vi "Initialization_channels.vi"(8 "error in (no error)":errorcluster, 9 "productNum":u32, 10 "vendorNum":u32, 11 "Device Item Ref in":T3 format="%.0x") -> (0 "error out":errorcluster, 2 "PAR":T1={"Loop time"={"Loop Rate"=5, "Processor"=-2}, "COM"={"COM IP"="192.168.8.70", "COM port"=30005, "Local port"=5556, "Next_IP 1"=0, "Next_IP 2"=0, "Next_IP 3"=0, "Next_IP 4"=0}, "O2Sensor1"={"Lambda"={"LSU4.2 Lambda"=[], "LSU4.2 Ip"=[], "LSU4.9 Lambda"=[], "LSU4.9 Ip"=[], "LZA03 Lambda"=[], "LZA03 Ip"=[], "LZA08 Lambda"=[], "LZA08 Ip"=[], "Custom Lambda"=[], "Custom Ip"=[]}, "Temp"={"LSU4.2 Temp"=[], "LSU4.2 Ohm"=[], "LSU4.9 Temp"=[], "LSU4.9 Ohm"=[], "LZA03 Temp"=[], "LZA03 Ohm"=[], "LZA08 Temp"=[], "LZA08 Ohm"=[], "Custom Temp"=[], "Custom Ohm"=[]}, "Lambda Type"=0, "PID"={"Ki"=0.0, "Kp"=0.0, "Kd"=0.0, "FeedFW"=0.0}}, "O2Sensor2"={"Lambda"={"LSU4.2 Lambda"=[], "LSU4.2 Ip"=[], "LSU4.9 Lambda"=[], "LSU4.9 Ip"=[], "LZA03 Lambda"=[], "LZA03 Ip"=[], "LZA08 Lambda"=[], "LZA08 Ip"=[], "Custom Lambda"=[], "Custom Ip"=[]}, "Temp"={"LSU4.2 Temp"=[], "LSU4.2 Ohm"=[], "LSU4.9 Temp"=[], "LSU4.9 Ohm"=[], "LZA03 Temp"=[], "LZA03 Ohm"=[], "LZA08 Temp"=[], "LZA08 Ohm"=[], "Custom Temp"=[], "Custom Ohm"=[]}, "Lambda Type"=0, "PID"={"Ki"=0.0, "Kp"=0.0, "Kd"=0.0, "FeedFW"=0.0}}, "O2Sensor3"={"Lambda"={"LSU4.2 Lambda"=[], "LSU4.2 Ip"=[], "LSU4.9 Lambda"=[], "LSU4.9 Ip"=[], "LZA03 Lambda"=[], "LZA03 Ip"=[], "LZA08 Lambda"=[], "LZA08 Ip"=[], "Custom Lambda"=[], "Custom Ip"=[]}, "Temp"={"LSU4.2 Temp"=[], "LSU4.2 Ohm"=[], "LSU4.9 Temp"=[], "LSU4.9 Ohm"=[], "LZA03 Temp"=[], "LZA03 Ohm"=[], "LZA08 Temp"=[], "LZA08 Ohm"=[], "Custom Temp"=[], "Custom Ohm"=[]}, "Lambda Type"=0, "PID"={"Ki"=0.0, "Kp"=0.0, "Kd"=0.0, "FeedFW"=0.0}}, "O2Sensor4"={"Lambda"={"LSU4.2 Lambda"=[], "LSU4.2 Ip"=[], "LSU4.9 Lambda"=[], "LSU4.9 Ip"=[], "LZA03 Lambda"=[], "LZA03 Ip"=[], "LZA08 Lambda"=[], "LZA08 Ip"=[], "Custom Lambda"=[], "Custom Ip"=[]}, "Temp"={"LSU4.2 Temp"=[], "LSU4.2 Ohm"=[], "LSU4.9 Temp"=[], "LSU4.9 Ohm"=[], "LZA03 Temp"=[], "LZA03 Ohm"=[], "LZA08 Temp"=[], "LZA08 Ohm"=[], "Custom Temp"=[], "Custom Ohm"=[]}, "Lambda Type"=0, "PID"={"Ki"=0.0, "Kp"=0.0, "Kd"=0.0, "FeedFW"=0.0}}, "Board"=1, "Mode"=enum."SLSC Mode", "vendor.Num"=4141, "product.Num"=0} {"Board" items=["ALMA-10201", "ALMA-10401"]; "O2Sensor4"."Lambda Type" items=["LSU4.2", "LSU4.9", "LZA03", "LZA08", "Custom", "[mA]"]; "O2Sensor3"."Lambda Type" items=["LSU4.2", "LSU4.9", "LZA03", "LZA08", "Custom", "[mA]"]; "O2Sensor2"."Lambda Type" items=["LSU4.2", "LSU4.9", "LZA03", "LZA08", "Custom", "[mA]"]; "O2Sensor1"."Lambda Type" items=["LSU4.2", "LSU4.9", "LZA03", "LZA08", "Custom", "[mA]"]}, 3 "Device Item Ref out":T3 format="%.0x")   [LabVIEW 2017, in "ALMA_10201-10401_O2SensorSim System Explorer.lvlib"]
uses:
  ALMA_10201-10401_O2SensorSim System Explorer.lvlib
  <vilib>/NI Veristand/Custom Device API/Custom Device Item Ref.ctl
  Engine/Par.ctl
  Engine/LambdaType.ctl
  <vilib>/NI Veristand/Custom Device API/Custom Device Channel.ctl
  <vilib>/NI Veristand/Custom Device API/Custom Device Channel Type.ctl
  <vilib>/NI Veristand/Custom Device API/Set Item Property (String).vi
  <vilib>/NI Veristand/Custom Device API/Get Item Property (String).vi
  Shared/Constants.vi
  <vilib>/NI Veristand/Custom Device API/Custom Device API.lvlib
  Shared/ALMA_10201-10401_O2SensorSim Shared.lvlib
panel:
  in  "Status":string[](array[string])=["SLSC Mod Update Rate", "SLSC Mod Loop Rate", "SLSC Mod Error Number"]
  in  "Status description":string[](array[string])=["", "", ""]
  in  "par 3":T1={"Loop time"={"Loop Rate"=0, "Processor"=0}, "COM"={"COM IP"="0.0.0.0", "COM port"=1, "Local port"=0, "Next_IP 1"=0, "Next_IP 2"=0, "Next_IP 3"=0, "Next_IP 4"=0}, "O2Sensor1"={"Lambda"={"LSU4.2 Lambda"=[], "LSU4.2 Ip"=[], "LSU4.9 Lambda"=[], "LSU4.9 Ip"=[], "LZA03 Lambda"=[], "LZA03 Ip"=[], "LZA08 Lambda"=[], "LZA08 Ip"=[], "Custom Lambda"=[], "Custom Ip"=[]}, "Temp"={"LSU4.2 Temp"=[], "LSU4.2 Ohm"=[], "LSU4.9 Temp"=[], "LSU4.9 Ohm"=[], "LZA03 Temp"=[], "LZA03 Ohm"=[], "LZA08 Temp"=[], "LZA08 Ohm"=[], "Custom Temp"=[], "Custom Ohm"=[]}, "Lambda Type"=0, "PID"={"Ki"=0.0, "Kp"=0.0, "Kd"=0.0, "FeedFW"=0.0}}, "O2Sensor2"={"Lambda"={"LSU4.2 Lambda"=[], "LSU4.2 Ip"=[], "LSU4.9 Lambda"=[], "LSU4.9 Ip"=[], "LZA03 Lambda"=[], "LZA03 Ip"=[], "LZA08 Lambda"=[], "LZA08 Ip"=[], "Custom Lambda"=[], "Custom Ip"=[]}, "Temp"={"LSU4.2 Temp"=[], "LSU4.2 Ohm"=[], "LSU4.9 Temp"=[], "LSU4.9 Ohm"=[], "LZA03 Temp"=[], "LZA03 Ohm"=[], "LZA08 Temp"=[], "LZA08 Ohm"=[], "Custom Temp"=[], "Custom Ohm"=[]}, "Lambda Type"=0, "PID"={"Ki"=0.0, "Kp"=0.0, "Kd"=0.0, "FeedFW"=0.0}}, "O2Sensor3"={"Lambda"={"LSU4.2 Lambda"=[], "LSU4.2 Ip"=[], "LSU4.9 Lambda"=[], "LSU4.9 Ip"=[], "LZA03 Lambda"=[], "LZA03 Ip"=[], "LZA08 Lambda"=[], "LZA08 Ip"=[], "Custom Lambda"=[], "Custom Ip"=[]}, "Temp"={"LSU4.2 Temp"=[], "LSU4.2 Ohm"=[], "LSU4.9 Temp"=[], "LSU4.9 Ohm"=[], "LZA03 Temp"=[], "LZA03 Ohm"=[], "LZA08 Temp"=[], "LZA08 Ohm"=[], "Custom Temp"=[], "Custom Ohm"=[]}, "Lambda Type"=0, "PID"={"Ki"=0.0, "Kp"=0.0, "Kd"=0.0, "FeedFW"=0.0}}, "O2Sensor4"={"Lambda"={"LSU4.2 Lambda"=[], "LSU4.2 Ip"=[], "LSU4.9 Lambda"=[], "LSU4.9 Ip"=[], "LZA03 Lambda"=[], "LZA03 Ip"=[], "LZA08 Lambda"=[], "LZA08 Ip"=[], "Custom Lambda"=[], "Custom Ip"=[]}, "Temp"={"LSU4.2 Temp"=[], "LSU4.2 Ohm"=[], "LSU4.9 Temp"=[], "LSU4.9 Ohm"=[], "LZA03 Temp"=[], "LZA03 Ohm"=[], "LZA08 Temp"=[], "LZA08 Ohm"=[], "Custom Temp"=[], "Custom Ohm"=[]}, "Lambda Type"=0, "PID"={"Ki"=0.0, "Kp"=0.0, "Kd"=0.0, "FeedFW"=0.0}}, "Board"=0, "Mode"=enum."SLSC Mode", "vendor.Num"=4141, "product.Num"=0} {"Board" items=["O2Sim_2ch", "O2Sim_4ch"]; "O2Sensor4"."Lambda Type" items=["LSU4.2", "LSU4.9", "LZA03", "LZA08", "Custom", "[mA]"]; "O2Sensor3"."Lambda Type" items=["LSU4.2", "LSU4.9", "LZA03", "LZA08", "Custom", "[mA]"]; "O2Sensor2"."Lambda Type" items=["LSU4.2", "LSU4.9", "LZA03", "LZA08", "Custom", "[mA]"]; "O2Sensor1"."Lambda Type" items=["LSU4.2", "LSU4.9", "LZA03", "LZA08", "Custom", "[mA]"]}
  in  "Setpoint":string[](array[string])=["Enable", "Lambda Target", "Sensor Temperature"]
  in  "Setpoint UOM":string[](array[string])=["", "", "°"]
  in  "Setpoint description":string[](array[string])=["Enable channel", "Lambda value setpoint", "Sensor temperature setpoint"]
  in  "Feedback":string[](array[string])=["Lambda Feedback", "Status", "Duty Cycle Heater", "Frequency Heater", "Ip", "Ri", "V_Ip", "V_Ri"]
  in  "Feedback UOM":string[](array[string])=["", "", "%", "Hz", "mA", "Ohm", "V", "V"]
  in  "Feedback Description":string[](array[string])=["Lambda feedback", "Sensor fault status", "Duty cycle heater feedback", "Frequency heater feedback", "Pumping current setpoint", "Resistance setpoint", "Analog setpoint to Ip_1", "Analog setpoint to Ri_1"]
  in  "Additional Control":string[](array[string])=["PID#", "Ki", "Kp", "Kd", "FF"]
  in  "Additional Control description":string[](array[string])=["Sensor selector for PID tuning", "PID integral coefficient", "PID proportional coefficient", "PID derivative coefficient", "Feed forward coefficient"]
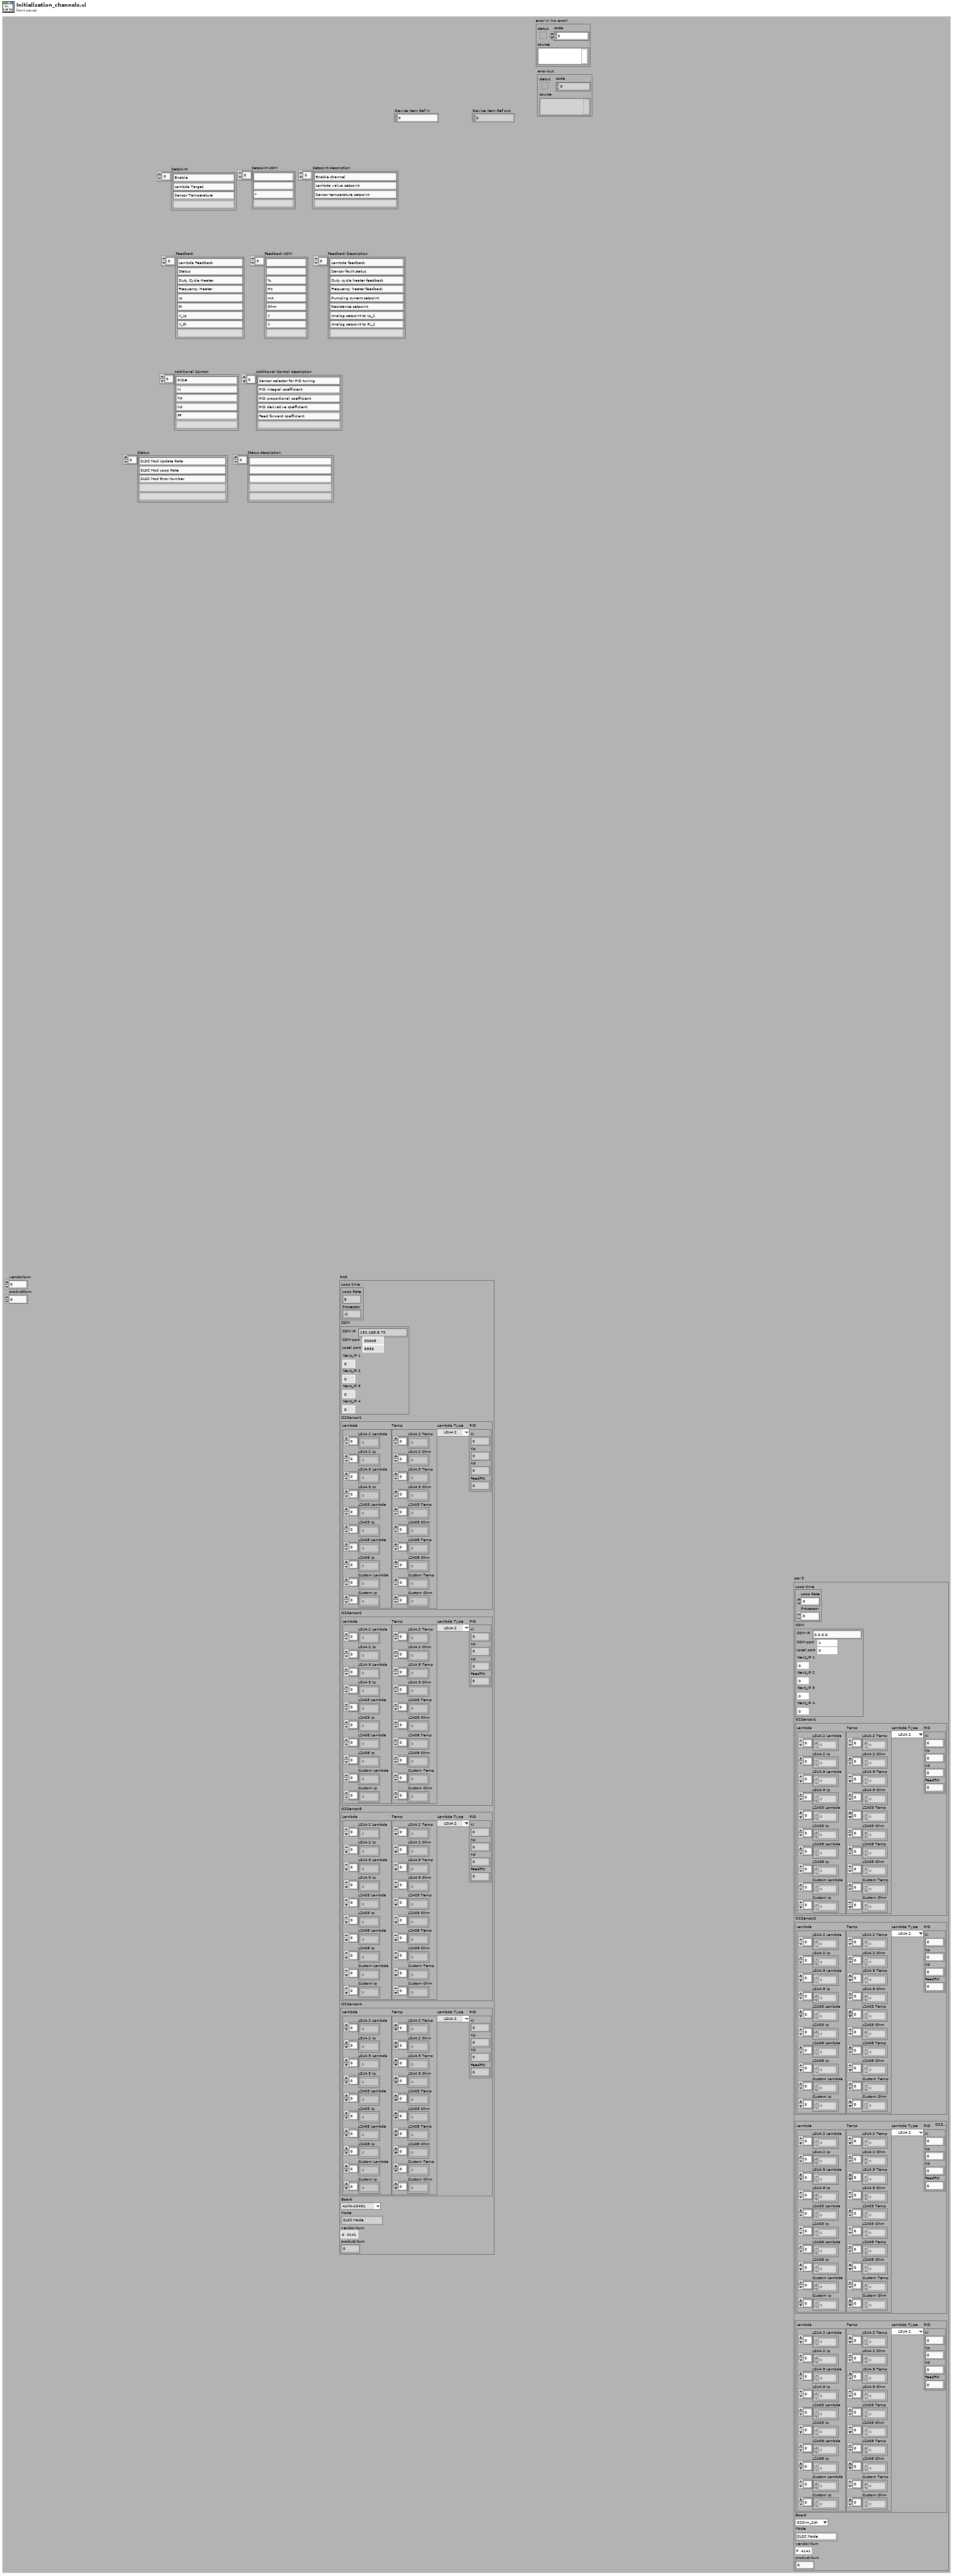
[diagram p1: front panel]
types:
  T1 = typedef "Par.ctl" = cluster{"Loop time":cluster{"Loop Rate":i64, "Processor":i32}, "COM":cluster{"COM IP":string, "COM port":u64, "Local port":u64, "Next_IP 1":u32, "Next_IP 2":u32, "Next_IP 3":u32, "Next_IP 4":u32}, "O2Sensor1":cluster{"Lambda":cluster{"LSU4.2 Lambda":dbl[], "LSU4.2 Ip":dbl[], "LSU4.9 Lambda":dbl[], "LSU4.9 Ip":dbl[], "LZA03 Lambda":dbl[], "LZA03 Ip":dbl[], "LZA08 Lambda":dbl[], "LZA08 Ip":dbl[], "Custom Lambda":dbl[], "Custom Ip":dbl[]}, "Temp":cluster{"LSU4.2 Temp":dbl[], "LSU4.2 Ohm":dbl[], "LSU4.9 Temp":dbl[], "LSU4.9 Ohm":dbl[], "LZA03 Temp":dbl[], "LZA03 Ohm":dbl[], "LZA08 Temp":dbl[], "LZA08 Ohm":dbl[], "Custom Temp":dbl[], "Custom Ohm":dbl[]}, "Lambda Type":T2, "PID":cluster{"Ki":dbl, "Kp":dbl, "Kd":dbl, "FeedFW":dbl}}, "O2Sensor2":cluster{"Lambda":cluster{"LSU4.2 Lambda":dbl[], "LSU4.2 Ip":dbl[], "LSU4.9 Lambda":dbl[], "LSU4.9 Ip":dbl[], "LZA03 Lambda":dbl[], "LZA03 Ip":dbl[], "LZA08 Lambda":dbl[], "LZA08 Ip":dbl[], "Custom Lambda":dbl[], "Custom Ip":dbl[]}, "Temp":cluster{"LSU4.2 Temp":dbl[], "LSU4.2 Ohm":dbl[], "LSU4.9 Temp":dbl[], "LSU4.9 Ohm":dbl[], "LZA03 Temp":dbl[], "LZA03 Ohm":dbl[], "LZA08 Temp":dbl[], "LZA08 Ohm":dbl[], "Custom Temp":dbl[], "Custom Ohm":dbl[]}, "Lambda Type":T2, "PID":cluster{"Ki":dbl, "Kp":dbl, "Kd":dbl, "FeedFW":dbl}}, "O2Sensor3":cluster{"Lambda":cluster{"LSU4.2 Lambda":dbl[], "LSU4.2 Ip":dbl[], "LSU4.9 Lambda":dbl[], "LSU4.9 Ip":dbl[], "LZA03 Lambda":dbl[], "LZA03 Ip":dbl[], "LZA08 Lambda":dbl[], "LZA08 Ip":dbl[], "Custom Lambda":dbl[], "Custom Ip":dbl[]}, "Temp":cluster{"LSU4.2 Temp":dbl[], "LSU4.2 Ohm":dbl[], "LSU4.9 Temp":dbl[], "LSU4.9 Ohm":dbl[], "LZA03 Temp":dbl[], "LZA03 Ohm":dbl[], "LZA08 Temp":dbl[], "LZA08 Ohm":dbl[], "Custom Temp":dbl[], "Custom Ohm":dbl[]}, "Lambda Type":T2, "PID":cluster{"Ki":dbl, "Kp":dbl, "Kd":dbl, "FeedFW":dbl}}, "O2Sensor4":cluster{"Lambda":cluster{"LSU4.2 Lambda":dbl[], "LSU4.2 Ip":dbl[], "LSU4.9 Lambda":dbl[], "LSU4.9 Ip":dbl[], "LZA03 Lambda":dbl[], "LZA03 Ip":dbl[], "LZA08 Lambda":dbl[], "LZA08 Ip":dbl[], "Custom Lambda":dbl[], "Custom Ip":dbl[]}, "Temp":cluster{"LSU4.2 Temp":dbl[], "LSU4.2 Ohm":dbl[], "LSU4.9 Temp":dbl[], "LSU4.9 Ohm":dbl[], "LZA03 Temp":dbl[], "LZA03 Ohm":dbl[], "LZA08 Temp":dbl[], "LZA08 Ohm":dbl[], "Custom Temp":dbl[], "Custom Ohm":dbl[]}, "Lambda Type":T2, "PID":cluster{"Ki":dbl, "Kp":dbl, "Kd":dbl, "FeedFW":dbl}}, "Board":u16, "Mode":enum16{"SLSC Mode", "ANALOG Mode"}, "vendor.Num":u32, "product.Num":u32}
  T2 = typedef "LambdaType.ctl" = u16
  T3 = typedef "Custom Device API.lvlib/Custom Device Item Ref.ctl" = u64
  T4 = typedef "Custom Device API.lvlib/Custom Device Channel.ctl" = cluster{"Type":T5, "Units":string, "Default Value":dbl, "Faultable":bool, "Scalable":bool}
  T5 = typedef "Custom Device API.lvlib/Custom Device Channel Type.ctl" = enum16{"Input", "Output"}
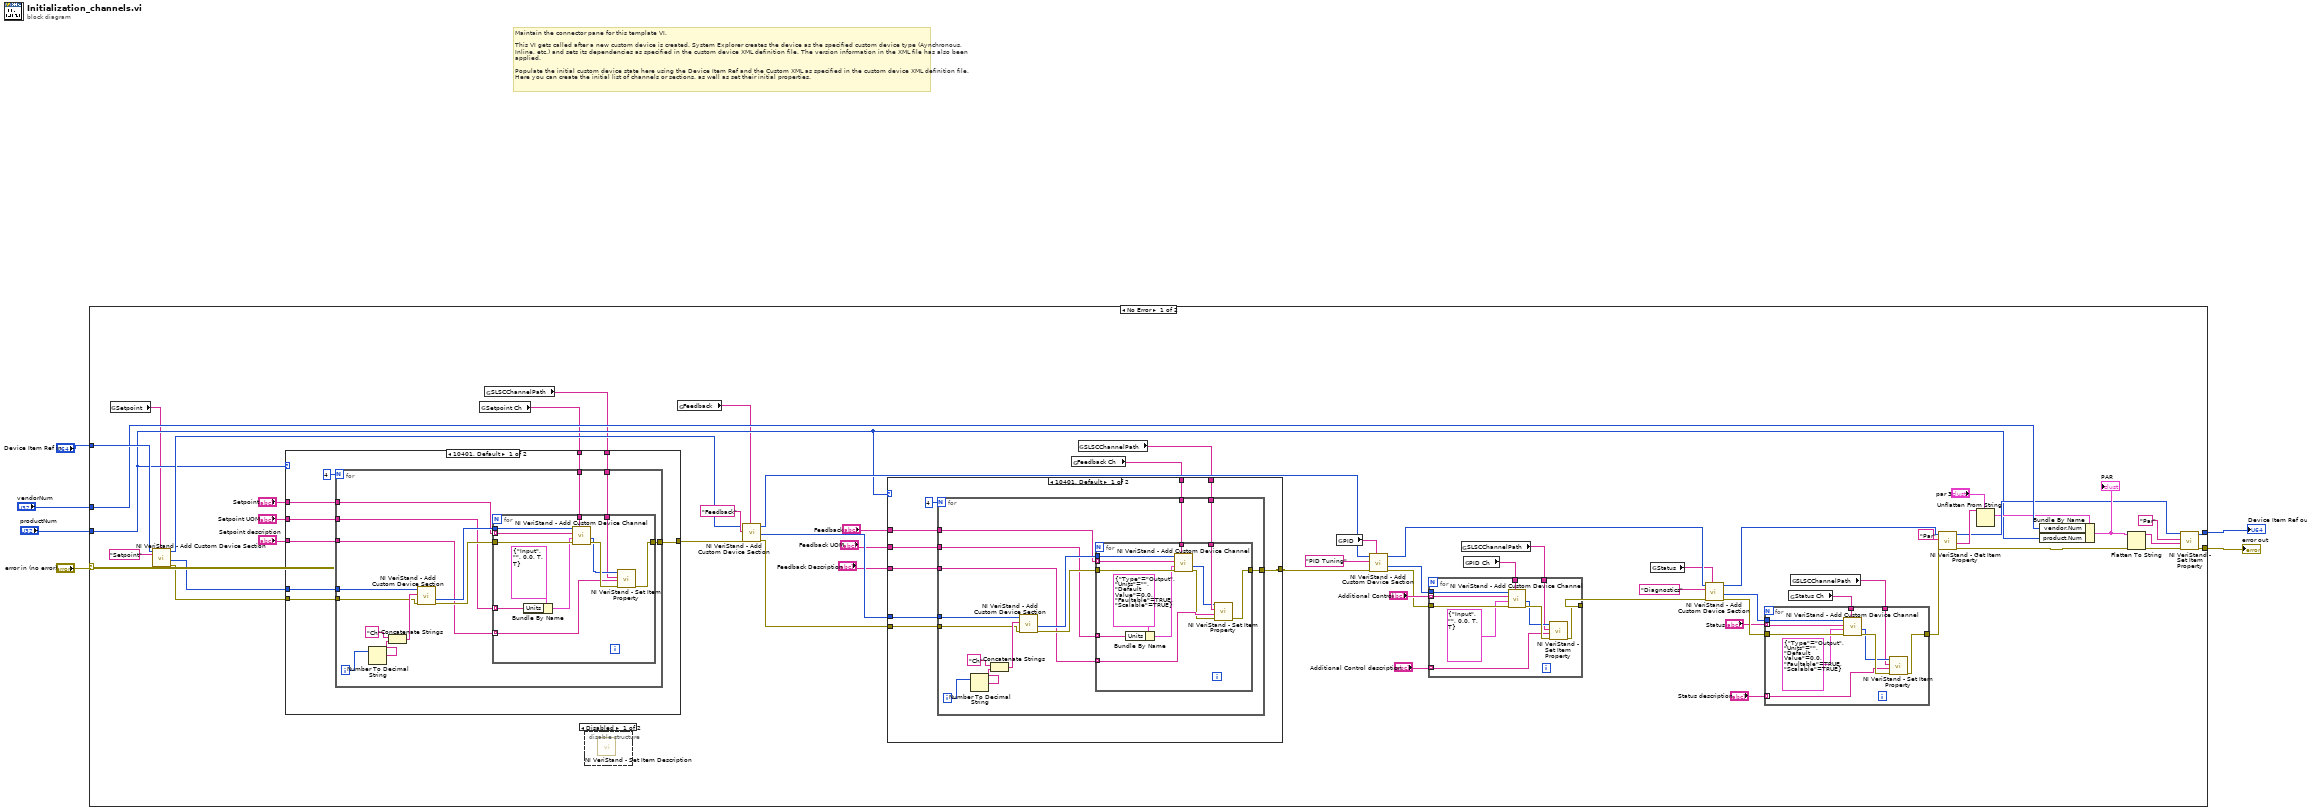
[diagram p0: block diagram]
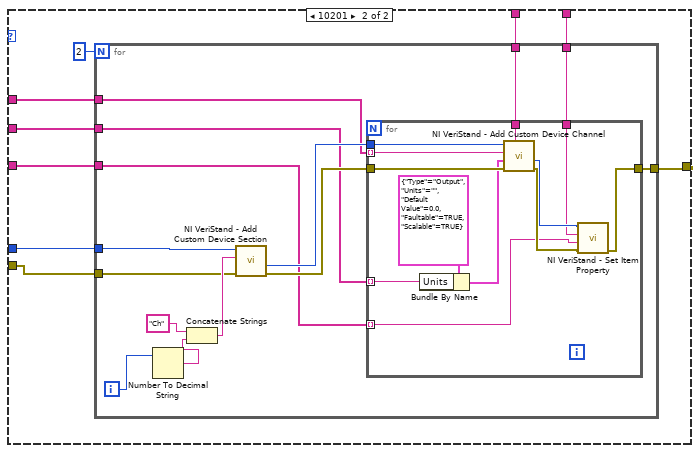
[diagram p3: hidden frame]
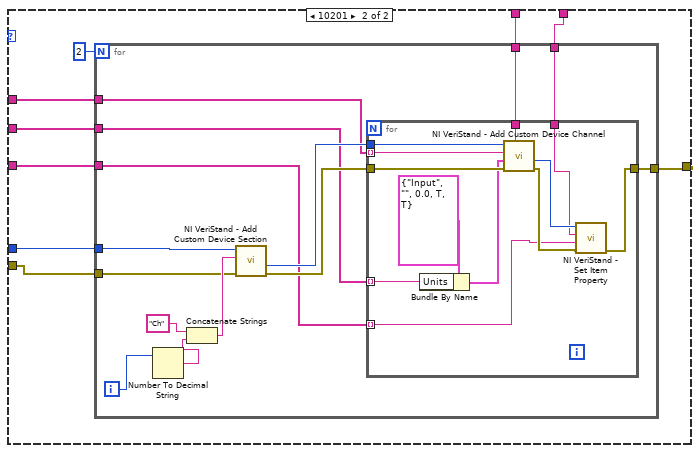
[diagram p4: hidden frame]
diagram:
  # "Maintain the connector pane for this template VI.\n\nThis VI gets called after a new custom device is created. System Explorer creates the device as the specified custom device type (Aynchronous, Inline, etc.) and sets its dependencies as specified in the custom device XML definition file. The version information in the XML file has also been applied.\n\nPopulate the initial custom device state here using the Device Item Ref and the Custom XML as specified in the custom device XML definition file. Here you can create the initial list of channels or sections, as well as set their initial properties."
  n1 = case shown="No Error" "error in (no error)" {
    selector: "error in (no error)" -> [w46 w226]
    tunnel: [w63 w226] -> w4
    tunnel: [w64 w225] -> w5
    tunnel: "Device Item Ref in" -> [w56 w225]
    tunnel: "vendorNum" -> [w54 _]
    tunnel: "productNum" -> [w34 _]
    frame No Error {
      n2 = global read "Constants.vi" "Setpoint"() -> (w8:string)
      n3 = call <vilib>:"NI VeriStand - Add Custom Device Section.vi"("GUID (Default Section)"=w8, "error in (no error)"=w46, "Section Name"="Setpoint", "Parent Ref in"=w56) -> ("error out"=w36:errorcluster, "Section Ptr"=w40:T3, "Parent Ref out"=w41:T3)  [unwired: 4 in, 1 out]
      n4 = global read "Constants.vi" "Setpoint Ch"() -> (w10:string)
      n5 = global read "Constants.vi" "SLSCChannelPath"() -> (w9:string)
      n6 = case shown="10401, Default" w34 {
        tunnel: w40 -> [w153 w188]
        tunnel: "Setpoint" -> [w151 w186]
        tunnel: "Setpoint UOM" -> [w150 w185]
        tunnel: "Setpoint description" -> [w149 w184]
        tunnel: [w148 w183] -> w35
        tunnel: w36 -> [w147 w182]
        tunnel: w10 -> [w146 w181]
        tunnel: w9 -> [w145 w180]
        frame 10401, Default {
          n7 = for {
            N: 4 -> [_]
            tunnel: w153 -> [w163]
            tunnel: w151 -> [w160]
            tunnel: w150 -> [w159]
            tunnel: w149 -> [w158]
            tunnel: [w157] -> w148
            tunnel: w147 -> [w156]
            tunnel: w146 -> [w155]
            tunnel: w145 -> [w154]
            i -> [w165]
            n8 = Number To Decimal String(number=w165) -> (decimal integer string=w167:string)  [unwired: 1 in]
            n9 = Concatenate Strings("Ch" ("Section Name"), w167) -> (w164:string)
            n10 = call <vilib>:"NI VeriStand - Add Custom Device Section.vi"("error in (no error)"=w156, "Section Name"=w164, "Parent Ref in"=w163) -> ("error out"=w161:errorcluster, "Section Ptr"=w162:T3)  [unwired: 5 in, 2 out]
            n11 = for {
              tunnel: w162 -> [w179]
              tunnel: w161 -> [w178]
              tunnel: [w171] -> w157
              tunnel: w160 -> [w177] mode=indexing
              tunnel: w159 -> [w175] mode=indexing
              tunnel: w158 -> [w168] mode=indexing
              tunnel: w155 -> [w173]
              tunnel: w154 -> [w169]
              n12 = Bundle By Name(cluster=T4 {"Type"=enum."Input", "Units"="", "Default Value"=0.0, "Faultable"=TRUE, "Scalable"=TRUE} ("Channel"), "Units"=w175) -> (w174:T4)
              n13 = call <vilib>:"NI VeriStand - Add Custom Device Channel.vi"("GUID (Default Channel)"=w173, "error in (no error)"=w178, "Channel"=w174, "Channel Name"=w177, "Parent Ref in"=w179) -> ("error out"=w172:errorcluster, "Channel Ref"=w170:T3)  [unwired: 3 in, 2 out]
              n14 = call-poly <vilib>:"NI VeriStand - Set Item Property.vi"("error in (no error)"=w172, "Value"=w168, "Property Name"=w169, "Item Ref in"=w170) -> ("error out"=w171:errorcluster)  [unwired: 5 in, 2 out]
            }
          }
        }
        frame 10201 {
          n15 = for {
            N: 2 -> [_]
            tunnel: w188 -> [w198]
            tunnel: w186 -> [w195]
            tunnel: w185 -> [w194]
            tunnel: w184 -> [w193]
            tunnel: [w192] -> w183
            tunnel: w182 -> [w191]
            tunnel: w181 -> [w190]
            tunnel: w180 -> [w189]
            i -> [w200]
            n16 = Number To Decimal String(number=w200) -> (decimal integer string=w202:string)  [unwired: 1 in]
            n17 = Concatenate Strings("Ch" ("Section Name"), w202) -> (w199:string)
            n18 = call <vilib>:"NI VeriStand - Add Custom Device Section.vi"("error in (no error)"=w191, "Section Name"=w199, "Parent Ref in"=w198) -> ("error out"=w196:errorcluster, "Section Ptr"=w197:T3)  [unwired: 5 in, 2 out]
            n19 = for {
              tunnel: w197 -> [w214]
              tunnel: w196 -> [w213]
              tunnel: [w206] -> w192
              tunnel: w195 -> [w212] mode=indexing
              tunnel: w194 -> [w210] mode=indexing
              tunnel: w193 -> [w203] mode=indexing
              tunnel: w190 -> [w208]
              tunnel: w189 -> [w204]
              n20 = Bundle By Name(cluster=T4 {"Type"=enum."Input", "Units"="", "Default Value"=0.0, "Faultable"=TRUE, "Scalable"=TRUE} ("Channel"), "Units"=w210) -> (w209:T4)
              n21 = call <vilib>:"NI VeriStand - Add Custom Device Channel.vi"("GUID (Default Channel)"=w208, "error in (no error)"=w213, "Channel"=w209, "Channel Name"=w212, "Parent Ref in"=w214) -> ("error out"=w207:errorcluster, "Channel Ref"=w205:T3)  [unwired: 3 in, 2 out]
              n22 = call-poly <vilib>:"NI VeriStand - Set Item Property.vi"("error in (no error)"=w207, "Value"=w203, "Property Name"=w204, "Item Ref in"=w205) -> ("error out"=w206:errorcluster)  [unwired: 5 in, 2 out]
            }
          }
        }
      }
      n23 = disable-structure shown="Disabled" {
        frame Disabled {
          n24 = call <vilib>:"NI VeriStand - Set Item Description.vi"() -> ()  [unwired: 3 in, 9 out]
        }
        frame Enabled {
        }
      }
      n25 = global read "Constants.vi" "Feedback"() -> (w7:string)
      n26 = call <vilib>:"NI VeriStand - Add Custom Device Section.vi"("GUID (Default Section)"=w7, "error in (no error)"=w35, "Section Name"="Feedback", "Parent Ref in"=w41) -> ("error out"=w33:errorcluster, "Section Ptr"=w32:T3, "Parent Ref out"=w42:T3)  [unwired: 4 in, 1 out]
      n27 = global read "Constants.vi" "Feedback Ch"() -> (w12:string)
      n28 = global read "Constants.vi" "SLSCChannelPath"() -> (w11:string)
      n29 = case shown="10401, Default" w34 {
        tunnel: w32 -> [w83 w118]
        tunnel: "Feedback" -> [w81 w116]
        tunnel: "Feedback UOM" -> [w80 w115]
        tunnel: "Feedback Description" -> [w79 w114]
        tunnel: [w78 w113] -> w28
        tunnel: w33 -> [w77 w112]
        tunnel: w12 -> [w76 w110]
        tunnel: w11 -> [w75 w111]
        frame 10401, Default {
          n30 = for {
            N: 4 -> [_]
            tunnel: w83 -> [w93]
            tunnel: w81 -> [w90]
            tunnel: w80 -> [w89]
            tunnel: w79 -> [w88]
            tunnel: [w87] -> w78
            tunnel: w77 -> [w86]
            tunnel: w76 -> [w85]
            tunnel: w75 -> [w84]
            i -> [w95]
            n31 = Number To Decimal String(number=w95) -> (decimal integer string=w97:string)  [unwired: 1 in]
            n32 = Concatenate Strings("Ch" ("Section Name"), w97) -> (w94:string)
            n33 = call <vilib>:"NI VeriStand - Add Custom Device Section.vi"("error in (no error)"=w86, "Section Name"=w94, "Parent Ref in"=w93) -> ("error out"=w91:errorcluster, "Section Ptr"=w92:T3)  [unwired: 5 in, 2 out]
            n34 = for {
              tunnel: w92 -> [w109]
              tunnel: w91 -> [w108]
              tunnel: [w102] -> w87
              tunnel: w90 -> [w107] mode=indexing
              tunnel: w89 -> [w105] mode=indexing
              tunnel: w88 -> [w100] mode=indexing
              tunnel: w85 -> [w103]
              tunnel: w84 -> [w101]
              n35 = Bundle By Name(cluster=T4 {"Type"=enum."Output", "Units"="", "Default Value"=0.0, "Faultable"=TRUE, "Scalable"=TRUE} ("Channel"), "Units"=w105) -> (w104:T4)
              n36 = call <vilib>:"NI VeriStand - Add Custom Device Channel.vi"("GUID (Default Channel)"=w103, "error in (no error)"=w108, "Channel"=w104, "Channel Name"=w107, "Parent Ref in"=w109) -> ("error out"=w99:errorcluster, "Channel Ref"=w98:T3)  [unwired: 3 in, 2 out]
              n37 = call-poly <vilib>:"NI VeriStand - Set Item Property.vi"("error in (no error)"=w99, "Value"=w100, "Property Name"=w101, "Item Ref in"=w98) -> ("error out"=w102:errorcluster)  [unwired: 5 in, 2 out]
            }
          }
        }
        frame 10201 {
          n38 = for {
            N: 2 -> [_]
            tunnel: w118 -> [w128]
            tunnel: w116 -> [w125]
            tunnel: w115 -> [w124]
            tunnel: w114 -> [w123]
            tunnel: [w122] -> w113
            tunnel: w112 -> [w121]
            tunnel: w111 -> [w120]
            tunnel: w110 -> [w119]
            i -> [w130]
            n39 = Number To Decimal String(number=w130) -> (decimal integer string=w132:string)  [unwired: 1 in]
            n40 = Concatenate Strings("Ch" ("Section Name"), w132) -> (w129:string)
            n41 = call <vilib>:"NI VeriStand - Add Custom Device Section.vi"("error in (no error)"=w121, "Section Name"=w129, "Parent Ref in"=w128) -> ("error out"=w126:errorcluster, "Section Ptr"=w127:T3)  [unwired: 5 in, 2 out]
            n42 = for {
              tunnel: w127 -> [w144]
              tunnel: w126 -> [w143]
              tunnel: [w137] -> w122
              tunnel: w125 -> [w142] mode=indexing
              tunnel: w124 -> [w140] mode=indexing
              tunnel: w123 -> [w135] mode=indexing
              tunnel: w120 -> [w134]
              tunnel: w119 -> [w133]
              n43 = Bundle By Name(cluster=T4 {"Type"=enum."Output", "Units"="", "Default Value"=0.0, "Faultable"=TRUE, "Scalable"=TRUE} ("Channel"), "Units"=w140) -> (w139:T4)
              n44 = call <vilib>:"NI VeriStand - Add Custom Device Channel.vi"("GUID (Default Channel)"=w133, "error in (no error)"=w143, "Channel"=w139, "Channel Name"=w142, "Parent Ref in"=w144) -> ("error out"=w138:errorcluster, "Channel Ref"=w136:T3)  [unwired: 3 in, 2 out]
              n45 = call-poly <vilib>:"NI VeriStand - Set Item Property.vi"("error in (no error)"=w138, "Value"=w135, "Property Name"=w134, "Item Ref in"=w136) -> ("error out"=w137:errorcluster)  [unwired: 5 in, 2 out]
            }
          }
        }
      }
      n46 = global read "Constants.vi" "PID"() -> (w15:string)
      n47 = call <vilib>:"NI VeriStand - Add Custom Device Section.vi"("GUID (Default Section)"=w15, "error in (no error)"=w28, "Section Name"="PID Tuning", "Parent Ref in"=w42) -> ("error out"=w57:errorcluster, "Section Ptr"=w47:T3, "Parent Ref out"=w20:T3)  [unwired: 4 in, 1 out]
      n48 = global read "Constants.vi" "SLSCChannelPath"() -> (w13:string)
      n49 = global read "Constants.vi" "PID Ch"() -> (w14:string)
      n50 = for {
        tunnel: w47 -> [w224]
        tunnel: w57 -> [w223]
        tunnel: [w219] -> w22
        tunnel: "Additional Control" -> [w222] mode=indexing
        tunnel: "Additional Control description" -> [w216] mode=indexing
        tunnel: w14 -> [w220]
        tunnel: w13 -> [w215]
        n51 = call <vilib>:"NI VeriStand - Add Custom Device Channel.vi"("GUID (Default Channel)"=w220, "error in (no error)"=w223, "Channel"=T4 {"Type"=enum."Input", "Units"="", "Default Value"=0.0, "Faultable"=TRUE, "Scalable"=TRUE}, "Channel Name"=w222, "Parent Ref in"=w224) -> ("error out"=w218:errorcluster, "Channel Ref"=w217:T3)  [unwired: 3 in, 2 out]
        n52 = call-poly <vilib>:"NI VeriStand - Set Item Property.vi"("error in (no error)"=w218, "Value"=w216, "Property Name"=w215, "Item Ref in"=w217) -> ("error out"=w219:errorcluster)  [unwired: 5 in, 2 out]
      }
      n53 = global read "Constants.vi" "Status"() -> (w18:string)
      n54 = call <vilib>:"NI VeriStand - Add Custom Device Section.vi"("GUID (Default Section)"=w18, "error in (no error)"=w22, "Section Name"="Diagnostics", "Parent Ref in"=w20) -> ("error out"=w25:errorcluster, "Section Ptr"=w26:T3, "Parent Ref out"=w19:T3)  [unwired: 4 in, 1 out]
      n55 = global read "Constants.vi" "Status Ch"() -> (w17:string)
      n56 = global read "Constants.vi" "SLSCChannelPath"() -> (w16:string)
      n57 = for {
        tunnel: w26 -> [w74]
        tunnel: w25 -> [w73]
        tunnel: [w68] -> w21
        tunnel: "Status" -> [w72] mode=indexing
        tunnel: "Status description" -> [w66] mode=indexing
        tunnel: w17 -> [w70]
        tunnel: w16 -> [w65]
        n58 = call <vilib>:"NI VeriStand - Add Custom Device Channel.vi"("GUID (Default Channel)"=w70, "error in (no error)"=w73, "Channel"=T4 {"Type"=enum."Output", "Units"="", "Default Value"=0.0, "Faultable"=TRUE, "Scalable"=TRUE}, "Channel Name"=w72, "Parent Ref in"=w74) -> ("error out"=w69:errorcluster, "Channel Ref"=w67:T3)  [unwired: 3 in, 2 out]
        n59 = call-poly <vilib>:"NI VeriStand - Set Item Property.vi"("error in (no error)"=w69, "Value"=w66, "Property Name"=w65, "Item Ref in"=w67) -> ("error out"=w68:errorcluster)  [unwired: 5 in, 2 out]
      }
      n60 = call-poly <vilib>:"NI VeriStand - Get Item Property.vi"("error in (no error)"=w21, "Property Name"="Par", "Item Ref in"=w19) -> ("error out"=w49:errorcluster, "Value"=w52:string, "Item Ref out"=w50:T3)  [unwired: 5 in, 1 out]
      n61 = Unflatten From String(type="par 3", binary string=w52) -> (value=w48:T1)  [unwired: 3 in, 2 out]
      n62 = Bundle By Name(cluster=w48, "vendor.Num"=w54, "product.Num"=w34) -> (w55:T1)
      "PAR" <- w55
      n63 = Flatten To String(anything=w55, error in (no error)=w49) -> (data string=w60:string, error out=w61:errorcluster)  [unwired: 2 in, 1 out]
      n64 = call-poly <vilib>:"NI VeriStand - Set Item Property.vi"("error in (no error)"=w61, "Value"=w60, "Property Name"="Par", "Item Ref in"=w50) -> ("error out"=w63:errorcluster, "Item Ref out"=w64:T3)  [unwired: 5 in, 1 out]
    }
    frame Error {
    }
  }
  "error out" <- w4
  "Device Item Ref out" <- w5
